vi "Teleop.vi"(10 "Match Info":T1={"Autonomous Elapsed Seconds"=0.0, "TeleOp Elapsed Seconds"=0.0, "Disabled Elapsed Seconds"=0.0, "Visited Autonomous"=FALSE, "Visited TeleOp"=FALSE, "Visited Disabled"=FALSE, "Autonomous Settings"={"Autonomous Style"=enum."Independent", "VI Refnum"=refnum}}, 11 "Call Context":T2) -> ()   [LabVIEW 2017]
doc: "This VI is called for each enabled TeleOp packet received from the DS. It is typically used to read from joysticks and other inputs and update I/O or setpoints for timed control loops. It should complete and return within 20 milliseconds or risk missing DS packets."
uses:
  <vilib>/Rock Robotics/WPI/DriverStation/WPI_DriverStationDerivedRobotMode.ctl
  <vilib>/Rock Robotics/WPI/DriverStation/WPI_DriverStationMatch Info.ctl
  <vilib>/Rock Robotics/WPI/Utilities/WPI_GetSetVariantRefNum.vi
  <vilib>/Rock Robotics/Network Tables/NT Write Boolean Array.vi
  <vilib>/Rock Robotics/Network Tables/NT Write Numeric Array.vi
panel:
  out "Lower Arm":bool
  out "Lift Arm":bool
  in  "Arm Rate":dbl=0.8
  in  "Turn Rate":dbl=0.5
  in  "Speed Rate":dbl=0.5
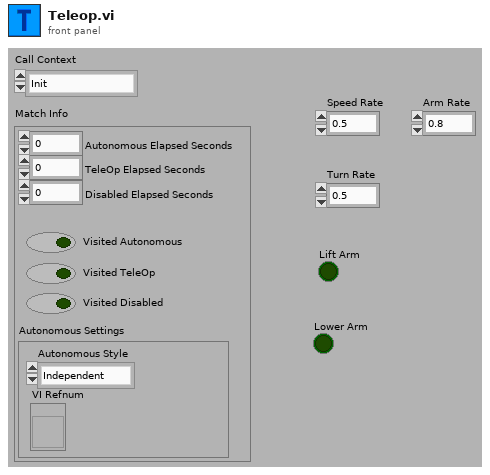
[diagram p1: front panel]
types:
  T1 = typedef "WPI_DriverStationMatch Info.ctl" = cluster{"Autonomous Elapsed Seconds":dbl, "TeleOp Elapsed Seconds":dbl, "Disabled Elapsed Seconds":dbl, "Visited Autonomous":bool, "Visited TeleOp":bool, "Visited Disabled":bool, "Autonomous Settings":cluster{"Autonomous Style":enum16{"Iterative", "Independent"}, "VI Refnum":refnum<vi>}}
  T2 = typedef "WPI_DriverStationDerivedRobotMode.ctl" = enum16{"Init", "Execute", "Stop"}
  T3 = typedef "WPI_JoystickDevRef.ctl" = cluster{"Device":T4}
  T4 = typedef "WPI_JoystickDeviceEnum.ctl" = enum16{"USB 0", "USB 1", "USB 2", "USB 3", "USB 4", "USB 5"}
  T5 = typedef "Command Status Info.ctl" = cluster{"Name":string, "Status":T6, "notifier out":T7}
  T6 = typedef "Completion Status.ctl" = enum16{"Successful", "Aborted", "Incomplete"}
  T7 = typedef "Completion Notifier.ctl" = refnum<notifier>
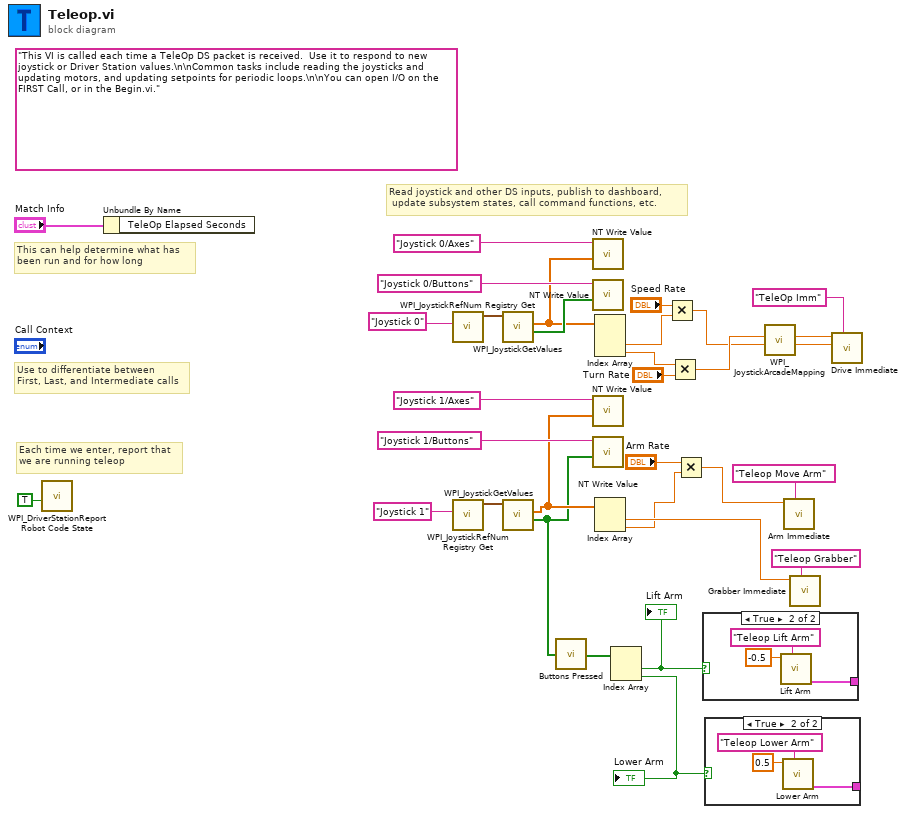
[diagram p0: block diagram]
diagram:
  (unwired) "This VI is called each time a TeleOp DS packet is received.  Use it to respond to new joystick or Driver Station values.\n\nCommon tasks include reading the joysticks and updating motors, and updating setpoints for periodic loops.\n\nYou can open I/O on the FIRST Call, or in the Begin.vi."
  # "Read joystick and other DS inputs, publish to dashboard,\n update subsystem states, call command functions, etc."
  # "Each time we enter, report that\nwe are running teleop"
  # "Use to differentiate between\nFirst, Last, and Intermediate calls"
  # "This can help determine what has\nbeen run and for how long"
  n1 = call <vilib>:"WPI_DriverStationReport Robot Code State.vi"("TeleOp"=TRUE ("Autonomous")) -> ()  [unwired: 10 in, 1 out]
  n2 = Unbundle By Name("Match Info") -> ()  [unwired: 1 out]
  n3 = call <vilib>:"WPI_JoystickRefNum Registry Get.vi"("refnum name"="Joystick 0") -> ("JoystickDevRef"=w29:T3)  [unwired: 1 in, 9 out]
  n4 = call <vilib>:"WPI_JoystickRefNum Registry Get.vi"("refnum name"="Joystick 1") -> ("JoystickDevRef"=w21:T3)  [unwired: 1 in, 9 out]
  n5 = call <vilib>:"WPI_JoystickGetValues.vi"("JoystickDevRef"=w29) -> ("Buttons"=w24:bool[], "Axes"=w23:dbl[])  [unwired: 6 in, 3 out]
  n6 = call <vilib>:"WPI_JoystickGetValues.vi"("JoystickDevRef"=w21) -> ("Buttons"=w1:bool[], "Axes"=w2:dbl[])  [unwired: 6 in, 3 out]
  n7 = call "Buttons Pressed.vi"("Button Values"=w1) -> ("Button Presses"=w7:bool[])
  n8 = call-poly <vilib>:"NT Write Value.vi"("Numeric Array"=w23, "Name"="Joystick 0/Axes") -> ()  [unwired: 9 in, 1 out]
  n9 = call-poly <vilib>:"NT Write Value.vi"("Boolean Array"=w24, "Name"="Joystick 0/Buttons") -> ()  [unwired: 9 in, 1 out]
  n10 = call-poly <vilib>:"NT Write Value.vi"("Numeric Array"=w2, "Name"="Joystick 1/Axes") -> ()  [unwired: 9 in, 1 out]
  n11 = call-poly <vilib>:"NT Write Value.vi"("Boolean Array"=w1, "Name"="Joystick 1/Buttons") -> ()  [unwired: 9 in, 1 out]
  n12 = Index Array(array=w23) -> (element #2=w14:dbl, element #3=w16:dbl)  [unwired: 3 in, 1 out]
  n13 = Index Array(array=w2) -> (element #1=w18:dbl, element #2=w9:dbl)  [unwired: 2 in]
  n14 = Index Array(array=w7) -> (element #1=w6:bool, element #2=w5:bool)  [unwired: 2 in]
  "Lift Arm" <- w6
  "Lower Arm" <- w5
  n15 = Multiply(x="Speed Rate", y=w14) -> (x*y=w13:dbl)
  n16 = Multiply(x=w16, y="Turn Rate") -> (x*y=w15:dbl)
  n17 = Multiply(x="Arm Rate", y=w9) -> (x*y=w8:dbl)
  n18 = case shown="True" w6 {
    tunnel: [_ w34] -> _
    frame False {
    }
    frame True {
      n19 = call "Lift Arm.vi"("Description"="Teleop Lift Arm", "Setpoint"=-0.5) -> ("Command Info Out"=w34:T5)  [unwired: 9 in]
    }
  }
  n20 = case shown="True" w5 {
    tunnel: [_ w37] -> _
    frame False {
    }
    frame True {
      n21 = call "Lower Arm.vi"("Description"="Teleop Lower Arm", "Setpoint"=0.5) -> ("Command Info Out"=w37:T5)  [unwired: 9 in]
    }
  }
  n22 = call <vilib>:"WPI_JoystickArcadeMapping.vi"("Y axis value"=w13, "X axis value"=w15) -> ("Right Motor Value"=w26:dbl, "Left Motor Value"=w27:dbl)  [unwired: 8 in]
  n23 = call "Arm Immediate.vi"("Description"="Teleop Move Arm", "Setpoint"=w8) -> ()  [unwired: 9 in, 1 out]
  n24 = call "Grabber Immediate.vi"("Description"="Teleop Grabber", "Setpoint"=w18) -> ()  [unwired: 9 in, 1 out]
  n25 = call "Drive Immediate.vi"("Description"="TeleOp Imm", "Right Setpoint"=w26, "Left Setpoint"=w27) -> ()  [unwired: 8 in, 1 out]
